vi "Dispense FN - ON - Setpoints (SubVI).vi"(0 "Main Concentration Setpoint (%)":dbl, 1 "Values IN":T1 {"Drain Time (s)" format="%.2f"; "Drain Rate (g/sec)" format="%.2f"}, 2 "Measured Mass (g)":dbl, 3 "Settings":T2={"ON Settings"={"Enable Dynamic Setpoint?"=TRUE, "Enable Dynamic Dispense Time?"=TRUE, "Enable Drain Rate Functions"=TRUE, "Dispense Sample Time (s)"=0.5, "Dispense Slope Ave"=0, "ON Timeout (sec)"=600.0, "1st Setpoint (% of Target)"=0.0, "2nd Setpoint (% of Target)"=0.0, "3rd Setpoint (% of Target)"=0.0, "Measure Dispense Delay (sec)"=0.0, "Settle Slope Sample Time (s)"=0.0}, "OFF Settings"={"Drain Sample Time (s)"=0.5, "Drain Rate Ave Size"=5, "Drain Rate Limits (± g/sec)"=10.0, "Level Slope Range (± g/sec)"=0.25, "OFF Timeout (sec)"=0.0, "Near SP Slope Level (± g/sec)"=0.01, "Near Setpoint Threshold (%)"=95.0}, "Overshoot Settings"={"Time Limit (s)"=60.0, "Container MAX (g)"=1500.0, "Max FILL Slope (+/- g/sec)"=10.0, "% Overshot to Enable (>)"=0.25}, "FILL Timeout (s)"=300.0, "Full Settle Time (s)"=3.0, "Pre-Hydrate \nSpray Time (s)"=10.0, "Pre-Hydrate \nWait Time (s)"=30.0}, 4 "State Change?":bool, 5 "Main Case Change?":bool) -> (15 "Values OUT":T1, 18 "Dynamic SP Valid?":bool, 19 "Enable Dispense Measure?":bool)   [LabVIEW 2009]
uses:
  <vilib>/ptbypt/NI_PtbyPt.lvlib
panel:
  # "Dispense Setpoints (SubVI)\nBlake Otting - October 2009"
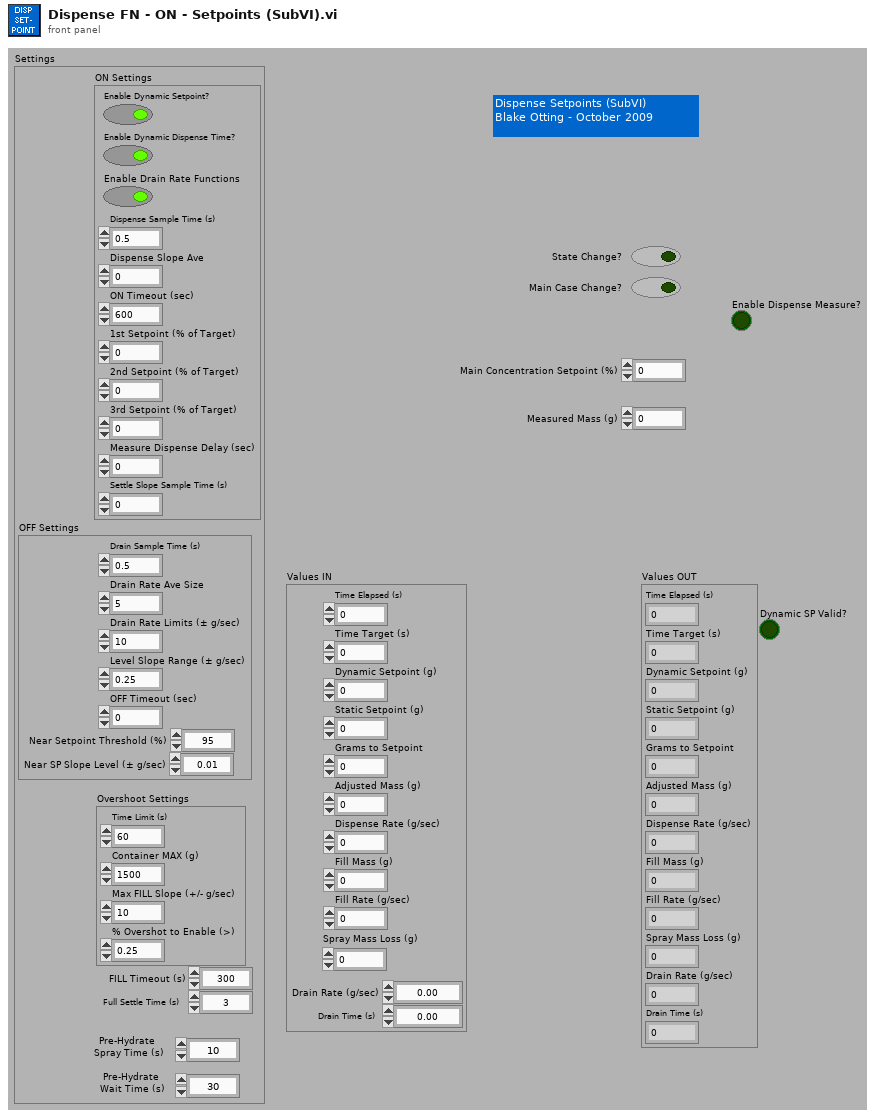
[diagram p1: front panel]
types:
  T1 = cluster{"Time Elapsed (s)":dbl, "Time Target (s)":dbl, "Dynamic Setpoint (g)":dbl, "Static Setpoint (g)":dbl, "Grams to Setpoint":dbl, "Adjusted Mass (g)":dbl, "Dispense Rate (g/sec)":dbl, "Fill Mass (g)":dbl, "Fill Rate (g/sec)":dbl, "Spray Mass Loss (g)":dbl, "Drain Rate (g/sec)":dbl, "Drain Time (s)":dbl}
  T2 = cluster{"ON Settings":cluster{"Enable Dynamic Setpoint?":bool, "Enable Dynamic Dispense Time?":bool, "Enable Drain Rate Functions":bool, "Dispense Sample Time (s)":dbl, "Dispense Slope Ave":i32, "ON Timeout (sec)":dbl, "1st Setpoint (% of Target)":dbl, "2nd Setpoint (% of Target)":dbl, "3rd Setpoint (% of Target)":dbl, "Measure Dispense Delay (sec)":dbl, "Settle Slope Sample Time (s)":dbl}, "OFF Settings":cluster{"Drain Sample Time (s)":dbl, "Drain Rate Ave Size":i32, "Drain Rate Limits (± g/sec)":dbl, "Level Slope Range (± g/sec)":dbl, "OFF Timeout (sec)":dbl, "Near SP Slope Level (± g/sec)":dbl, "Near Setpoint Threshold (%)":dbl}, "Overshoot Settings":cluster{"Time Limit (s)":dbl, "Container MAX (g)":dbl, "Max FILL Slope (+/- g/sec)":dbl, "% Overshot to Enable (>)":dbl}, "FILL Timeout (s)":dbl, "Full Settle Time (s)":dbl, "Pre-Hydrate \nSpray Time (s)":dbl, "Pre-Hydrate \nWait Time (s)":dbl}
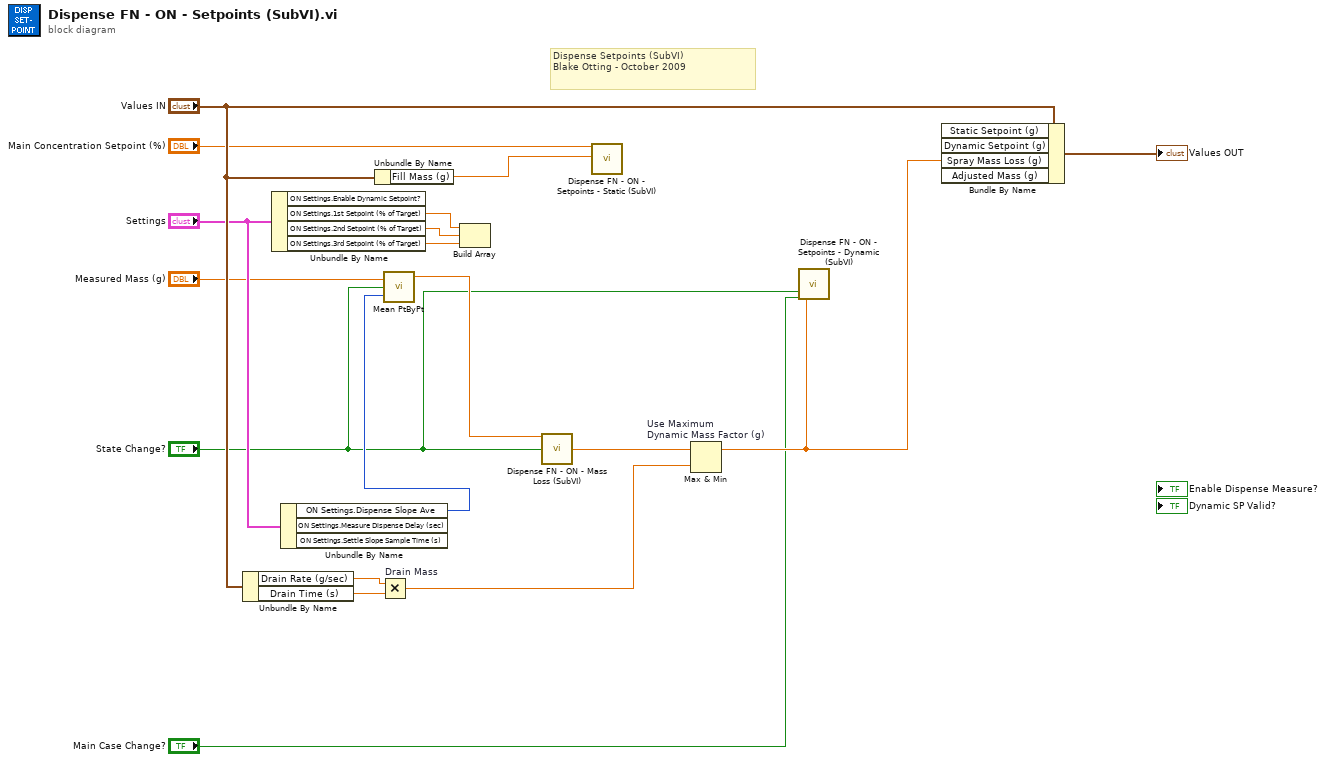
[diagram p0: block diagram]
diagram:
  # "Dispense Setpoints (SubVI)\nBlake Otting - October 2009"
  n1 = Unbundle By Name("Values IN") -> ("Drain Rate (g/sec)"=w18:dbl, "Drain Time (s)"=w17:dbl)
  n2 = Unbundle By Name("Settings") -> ("ON Settings.1st Setpoint (% of Target)"=w11:dbl, "ON Settings.2nd Setpoint (% of Target)"=w10:dbl, "ON Settings.3rd Setpoint (% of Target)"=w9:dbl)  [unwired: 1 out]
  n3 = Unbundle By Name("Settings") -> ("ON Settings.Dispense Slope Ave"=w4:i32)  [unwired: 2 out]
  n4 = Unbundle By Name("Values IN") -> ("Fill Mass (g)"=w15:dbl)
  n5 = Multiply "Drain Mass"(x=w18, y=w17) -> (x*y=w8:dbl)
  n6 = call <vilib>:"Mean PtByPt.vi"("x"="Measured Mass (g)", "sample length"=w4, "initialize"="State Change?") -> ("mean"=w5:dbl)  [unwired: 2 out]
  n7 = Build Array(w11, w10, w9) -> ()  [unwired: 1 out]
  n8 = call "Dispense FN - ON - Mass Loss (SubVI).vi"("Measured Mass (g)"=w5, "State Change?"="State Change?") -> ("Dispense Mass Loss"=w7:dbl)  [unwired: 3 in, 10 out]
  n9 = call "Dispense FN - ON - Setpoints - Static (SubVI).vi"("Main Concentration Setpoint (%)"="Main Concentration Setpoint (%)", 2:w15) -> ()  [unwired: 1 in, 17 out]
  n10 = Max & Min "Use Maximum\nDynamic Mass Factor (g)"(x=w7, y=w8) -> (max(x,y)=w12:dbl)  [unwired: 1 out]
  n11 = call "Dispense FN - ON - Setpoints - Dynamic (SubVI).vi"("State Change?"="State Change?", "Main Case Change?"="Main Case Change?", "Drain Mass Gain (g)"=w12) -> ()  [unwired: 10 in, 7 out]
  n12 = Bundle By Name(cluster="Values IN", "Spray Mass Loss (g)"=w12) -> (→"Values OUT":T1)  [unwired: 3 in]
